vi "Extract Phases from Phase-TTL data.vi"(3 "TTL row index":i32=1, 4 "Phase row index":i32, 5 "Phase-TTL Data":dbl[][](array[numeric])) -> (0 "Input TTL array":dbl[](array[numeric]), 1 "Input Phase Array":dbl[](array[numeric]), 2 "Extracted Phases":dbl[](array[numeric]))   [LabVIEW 2009]
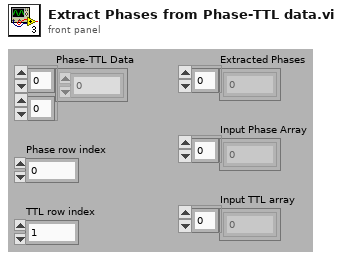
[diagram p1: front panel]
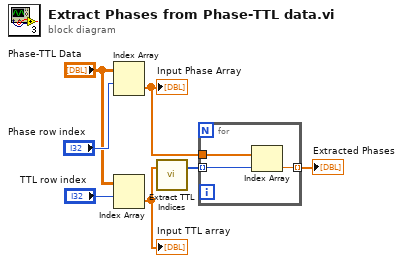
[diagram p0: block diagram]
diagram:
  n1 = Index Array(array="Phase-TTL Data", index (row)="Phase row index") -> (element=w6:dbl[])  [unwired: 1 in]
  "Input Phase Array" <- w6
  n2 = Index Array(array="Phase-TTL Data", index (row)="TTL row index") -> (element=w4:dbl[])  [unwired: 1 in]
  "Input TTL array" <- w4
  n3 = call "Extract TTL Indices.vi"("Analog TTL"=w4) -> ("Rising Transition Indices"=w5:u32[])  [unwired: 1 in, 1 out]
  n4 = for {
    tunnel: w5 -> [w10] mode=indexing
    tunnel: w6 -> [w9]
    tunnel: [w8] -> w7 mode=indexing
    n5 = Index Array(array=w9, index=w10) -> (element=w8:dbl)
  }
  "Extracted Phases" <- w7
